vi "BB_WPI_CameraDetermine Camera Type.vi"(10 "Port":string="1181") -> (2 "port":i32, 3 "address":string, 4 "cgi string":string, 5 "parameters":T1(array[cluster]))   [LabVIEW 2016]
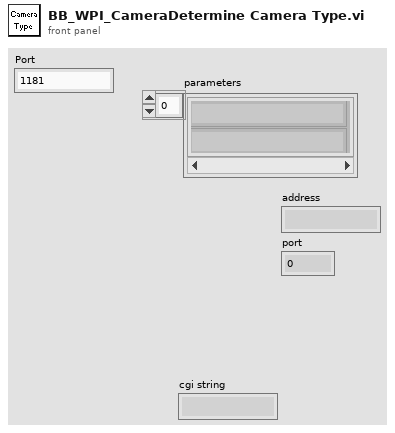
[diagram p1: front panel]
types:
  T1 = cluster{"token string":string, "token string 2":string}[]
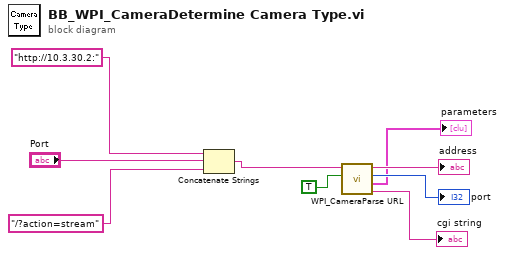
[diagram p0: block diagram]
diagram:
  n1 = Concatenate Strings("http://10.3.30.2:", "Port", "/?action=stream") -> (w4:string)
  n2 = call <vilib>:"WPI_CameraParse URL.vi"("Full"=TRUE, "URL"=w4) -> ("cgi string"=→"cgi string":string, "parameters"=→"parameters":T1, "port"=→"port":i32, "address"=→"address":string)  [unwired: 6 in]
